vi "IntersectLinePolys.vi"(10 "Line2D":T2, 11 "Polys":T3[](array[typedef])) -> (3 "Intersections":T1[](array[typedef]))   [LabVIEW 2014]
uses:
  TypeDefs/Poly2DwSlope.ctl
  TypeDefs/Point2DwSlope.ctl
  TypeDefs/Line2D.ctl
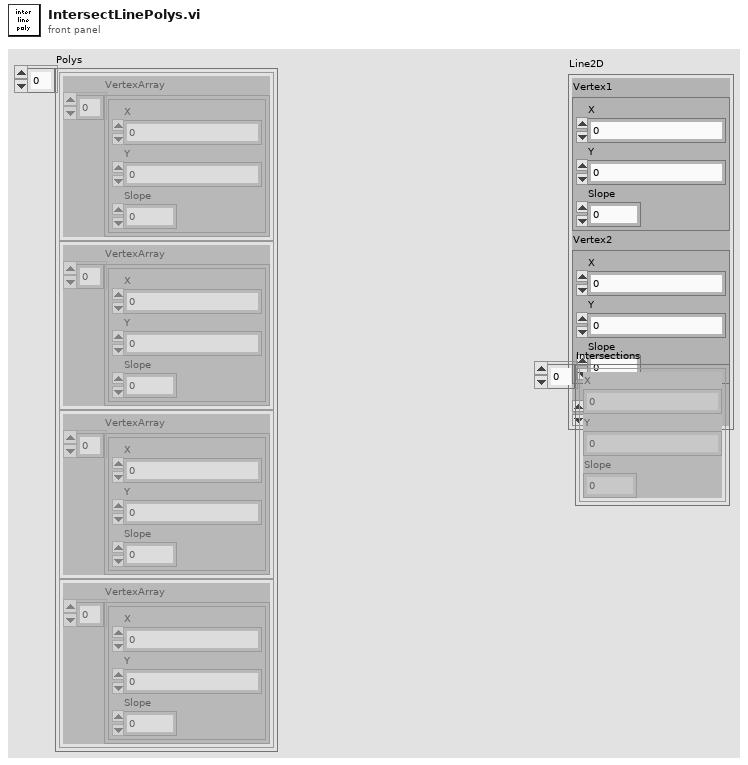
[diagram p1: front panel]
types:
  T1 = typedef "Point2DwSlope.ctl" = cluster{"X":sgl, "Y":sgl, "Slope":dbl}
  T2 = typedef "Line2D.ctl" = cluster{"Vertex1":T1, "Vertex2":T1, "Slope":dbl}
  T3 = typedef "Poly2DwSlope.ctl" = cluster{"VertexArray":T1[]}
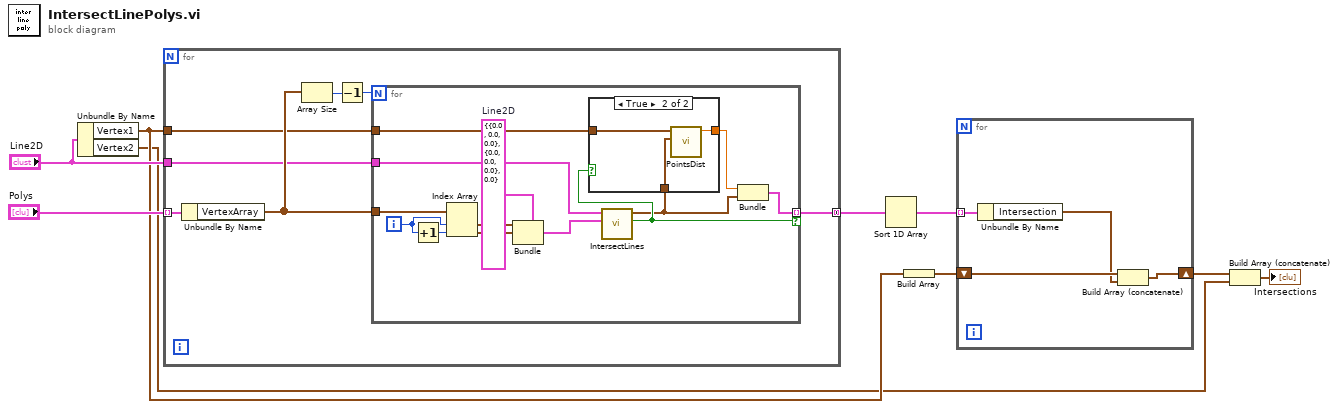
[diagram p0: block diagram]
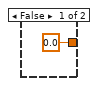
[diagram p2: hidden frame]
diagram:
  n1 = Unbundle By Name("Line2D") -> ("Vertex1"=w4:T1, "Vertex2"=w2:T1)
  n2 = for {
    tunnel: "Polys" -> [w14] mode=indexing
    tunnel: "Line2D" -> [w12]
    tunnel: w4 -> [w11]
    tunnel: [w10] -> w7 mode=concatenating
    n3 = Unbundle By Name(w14) -> ("VertexArray"=w13:T1[])
    n4 = Array Size(array=w13) -> (size(s)=w16:i32)
    n5 = Decrement(x=w16) -> (x-1=w15:i32)
    n6 = for {
      N: w15 -> [_]
      tunnel: w13 -> [w29]
      tunnel: w12 -> [w24]
      tunnel: [w18] -> w10 mode=indexing if=w21
      tunnel: w11 -> [w22]
      i -> [w27]
      w17 = T2 {"Vertex1"={"X"=0.0, "Y"=0.0, "Slope"=0.0}, "Vertex2"={"X"=0.0, "Y"=0.0, "Slope"=0.0}, "Slope"=0.0}  # Line2D
      n7 = Increment(x=w27) -> (x+1=w28:i32)
      n8 = Index Array(array=w29, index #1=w27, index #2=w28) -> (element #1=w26:T1, element #2=w25:T1)
      n9 = Bundle(cluster=w17, "Vertex1"=w26, "Vertex2"=w25) -> (w23:T2)  [unwired: 1 in]
      n10 = call "IntersectLines.vi"("Line2D_2"=w23, "Line2D_1"=w24) -> ("Intersect?"=w21:bool, "Intersection"=w19:T1)  [unwired: 8 in]
      n11 = case shown="True" w21 {
        tunnel: w22 -> [_ w33]
        tunnel: w19 -> [_ w32]
        tunnel: [sgl 0.0 ("Dist") w31] -> w20
        frame False {
        }
        frame True {
          n12 = call "PointsDist.vi"("Point2"=w32, "Point1"=w33) -> ("Dist"=w31:sgl)  [unwired: 9 in]
        }
      }
      n13 = Bundle("Dist"=w20, "Intersection"=w19) -> (w18:cluster{"Dist":sgl, "Intersection":T1})  [unwired: 1 in]
    }
  }
  n14 = Sort 1D Array(array=w7) -> (sorted array=w6:cluster{"Dist":sgl, "Intersection":T1}[])
  n15 = Build Array(w4) -> (w5:T1[])
  n16 = for {
    tunnel: w6 -> [w37] mode=indexing
    shift-right: [w35] -> w3
    shift-left: w5 -> [w36]
    n17 = Unbundle By Name(w37) -> ("Intersection"=w34:T1)
    n18 = Build Array (concatenate)(w36, w34) -> (w35:T1[])
  }
  n19 = Build Array (concatenate)(w3, w2) -> (→"Intersections":T1[])
